vi "Destruct.vi"(8 "error in (no error)":errorcluster, 11 "MagiQmw3 in":refnum<class "MagiQmw3.lvclass">) -> (0 "error out":errorcluster)   [LabVIEW 2012, in "MagiQmw3.lvclass"]
uses:
  MagiQmw3.lvclass
  MagiQmw3.lvclass/MagiQmw3.ctl
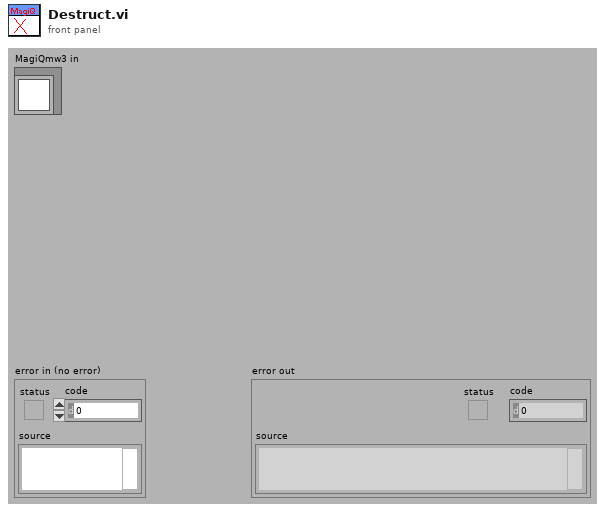
[diagram p1: front panel]
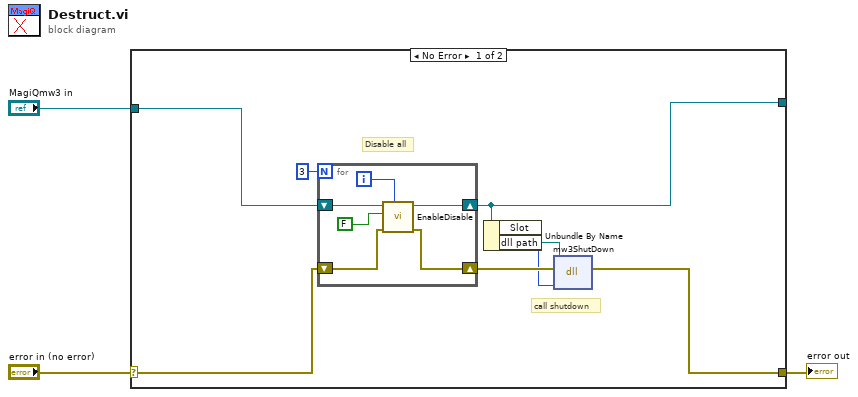
[diagram p0: block diagram]
diagram:
  n1 = case shown="No Error" "error in (no error)" {
    selector: "error in (no error)" -> [w9 w19]
    tunnel: [w4 w19] -> w1
    tunnel: "MagiQmw3 in" -> [w10 w18]
    tunnel: [w7 w18] -> _
    frame No Error {
      # "call shutdown"
      # "Disable all"
      n2 = for {
        N: 3 -> [_]
        shift-right: [w16] -> w7
        shift-left: w10 -> [w15]
        shift-right: [w12] -> w8
        shift-left: w9 -> [w13]
        i -> [w14]
        n3 = call "EnableDisable.vi"("ch"=w14, "error in (no error)"=w13, "Enable"=FALSE, "MagiQmw3 in"=w15) -> ("error out"=w12:errorcluster, "MagiQmw3 out"=w16:refnum<class "MagiQmw3.lvclass">)  [unwired: 6 in]
      }
      n4 = Unbundle By Name(w7) -> ("Slot"=w6:u16, "dll path"=w5:path)
      n5 = dll-call lib="PulserLib.dll" fn="mw3ShutDown"(path in=w5, error in=w8, "slot"=w6) -> (error out=w4:errorcluster)  [unwired: 3 in, 1 out]
    }
    frame Error {
    }
  }
  "error out" <- w1
